vi "stage_comp_z.vi"(11 "xpos":dbl=53.07 format="%#_13g") -> (3 "zcorr":dbl)   [LabVIEW 2018]
panel:
  in  "p 4":dbl=53.07 format="%#_13g"
  in  "p 3":dbl=-0.07201 format="%#_13g"
  in  "p 2":dbl=1.86e-05 format="%#_13g"
  in  "p1":dbl=-5.2e-10 format="%#_13g"
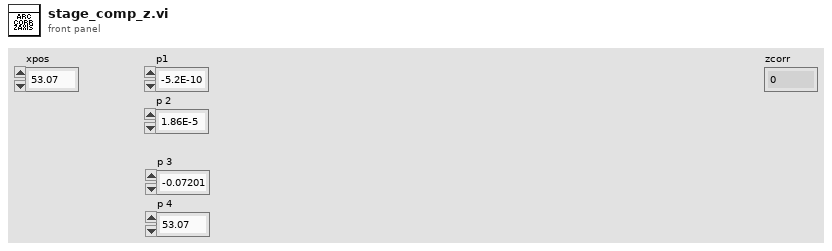
[diagram p1: front panel]
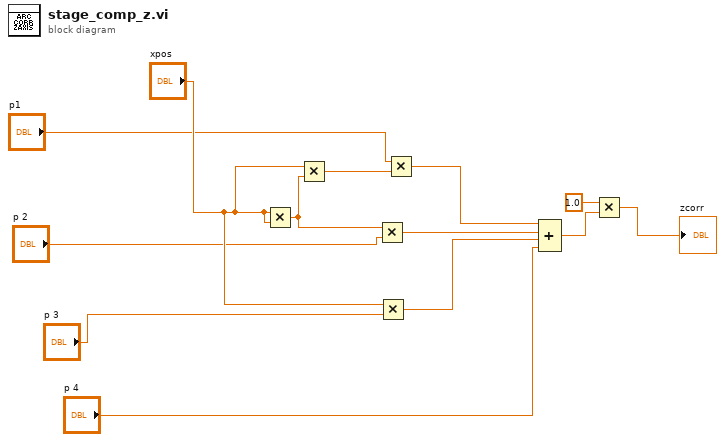
[diagram p0: block diagram]
diagram:
  n1 = Multiply(x="xpos", y="xpos") -> (x*y=w6:dbl)
  n2 = Multiply(x="xpos", y=w6) -> (x*y=w13:dbl)
  n3 = Multiply(x=w6, y="p 2") -> (x*y=w11:dbl)
  n4 = Multiply(x="xpos", y="p 3") -> (x*y=w10:dbl)
  n5 = Multiply(x="p1", y=w13) -> (x*y=w12:dbl)
  n6 = Compound Arithmetic op=ADD(w12, w11, w10, "p 4") -> (w2:dbl)
  n7 = Multiply(x=1.0, y=w2) -> (x*y=→"zcorr":dbl)
